vi "makeTIUnderlayPlotCommands.vi"(6 "plotInfoArray":T1(array[cluster]), 9 "Scale":dbl=300.0 caption="Scale 1:" min=1.0 max=10000.0 step=50.0) -> (1 "UnderlayPlotSeries":string[](array[string]), 2 "Pre-plot Injection":string)   [LabVIEW 2013]
uses:
  at.ctl
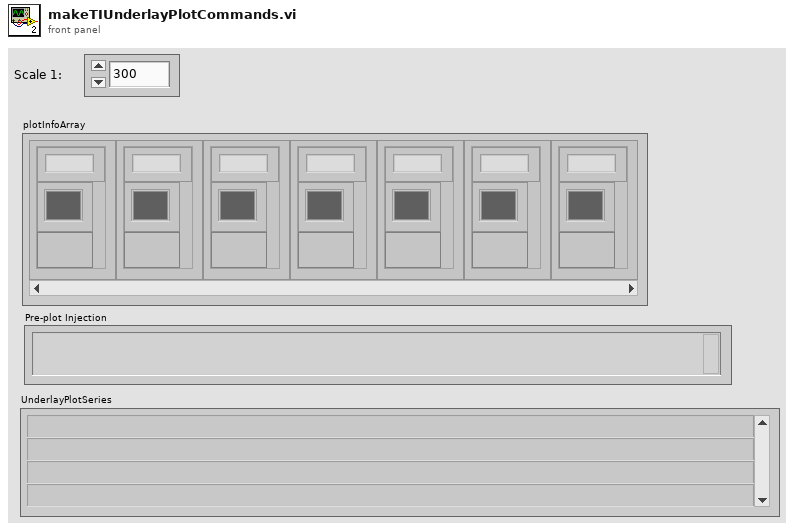
[diagram p1: front panel]
types:
  T1 = cluster{"Plot Name":string, "Plot.Plot Color":u32, "Plot.Visible?":bool}[]
  T2 = typedef "at.ctl" = cluster{"XcoordSys":string, "YcoordSys":string, "Xvalue":dbl, "Yvalue":dbl}
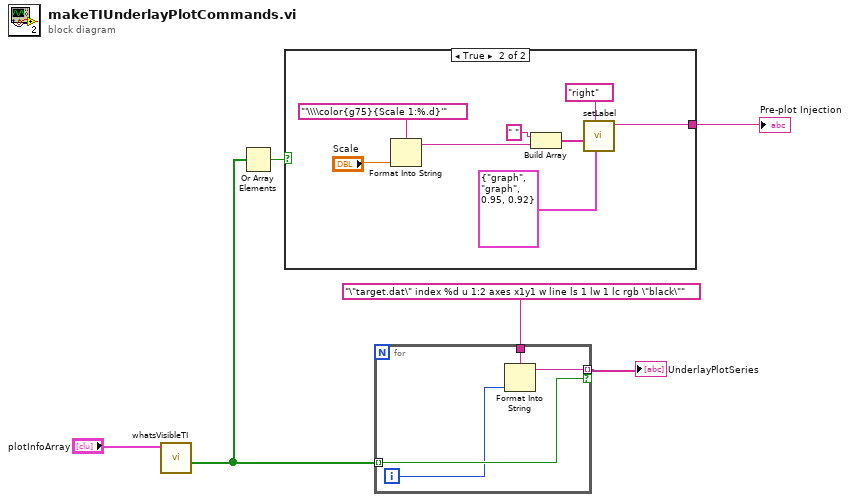
[diagram p0: block diagram]
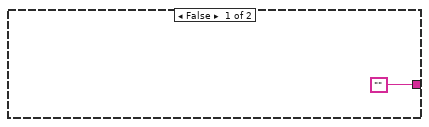
[diagram p2: hidden frame]
diagram:
  n1 = call "whatsVisibleTI.vi"("UplotInfoArray"="plotInfoArray") -> ("Targets Visible"=w3:bool[])  [unwired: 10 in]
  n2 = Or Array Elements(Boolean array=w3) -> (logical OR=w1:bool)
  n3 = case shown="True" w1 {
    tunnel: ["" w8] -> w2
    frame False {
    }
    frame True {
      n4 = Format Into String(format string="'\\\\color{g75}{Scale 1:%.d}'", "Scale") -> (resulting string=w15:string)  [unwired: 2 in, 1 out]
      n5 = Build Array(" " ("element"), w15) -> (w14:string[])
      n6 = call "setLabel.vi"("\"At\" location"=T2 {"XcoordSys"="graph", "YcoordSys"="graph", "Xvalue"=0.95, "Yvalue"=0.92} ("\"At\" location"), "Justify"="right", "multilineLabel"=w14) -> ("String out"=w8:string)  [unwired: 7 in, 1 out]
    }
  }
  "Pre-plot Injection" <- w2
  n7 = for {
    tunnel: [w19] -> w4 mode=indexing if=w18
    tunnel: w3 -> [w18] mode=indexing
    tunnel: "\"target.dat\" index %d u 1:2 axes x1y1 w line ls 1 lw 1 lc rgb \"black\"" ("String") -> [w17]
    i -> [w16]
    n8 = Format Into String(format string=w17, w16) -> (resulting string=w19:string)  [unwired: 2 in, 1 out]
  }
  "UnderlayPlotSeries" <- w4
